vi "Get Error Details from Error Cluster.vi"(11 "error":errorcluster) -> (1 "Message":string, 2 "Call Chain":string, 3 "Source":string)   [LabVIEW 2013, in "JUnit for Azure Pipelines.lvclass"]
uses:
  JUnit for Azure Pipelines.lvclass
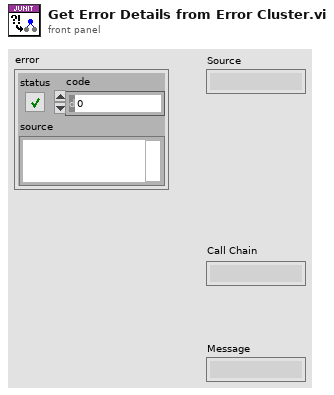
[diagram p1: front panel]
types:
  T1 = typedef "TagReturnType.ctl" = enum16{"No Tag", "<err>", "<append>"}
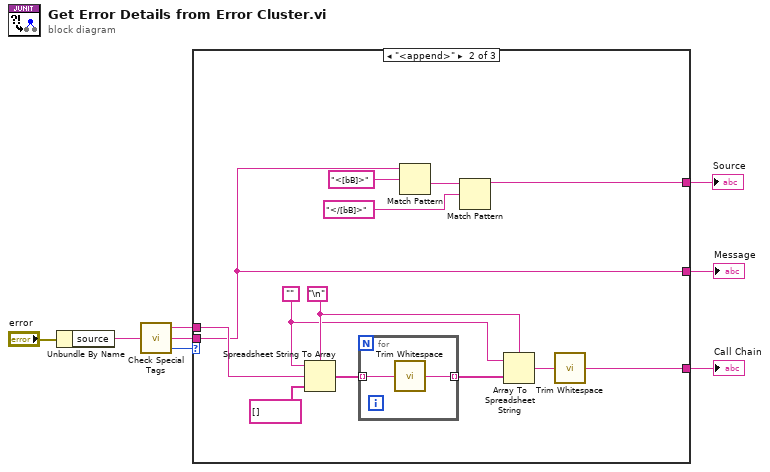
[diagram p0: block diagram]
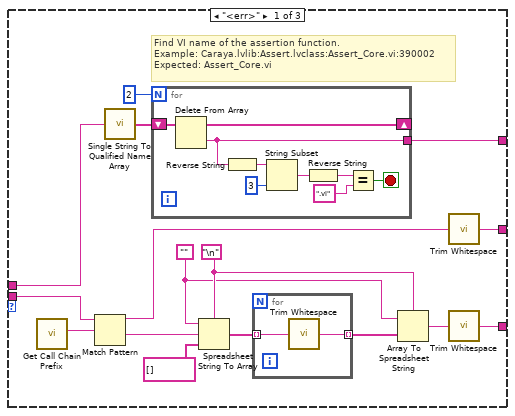
[diagram p2: hidden frame]
diagram:
  n1 = Unbundle By Name("error") -> ("source"=w1:string)
  n2 = call <vilib>:"Check Special Tags.vi"("source"=w1) -> ("Before Tag (source)"=w4:string, "After Tag (special data)"=w6:string, "Tag Found?"=w2:T1)
  n3 = case shown="\"<append>\"" w2 {
    tunnel: [w18 w41 _] -> w8
    tunnel: w6 -> [w17 w36 _]
    tunnel: [w13 w36 _] -> w5
    tunnel: w4 -> [w12 w42 _]
    tunnel: [w9 w37 _] -> w3
    frame "<err>" {
      w19 = ""
      w20 = "\n"
      # "Find VI name of the assertion function.\nExample: Caraya.lvlib:Assert.lvclass:Assert_Core.vi:390002\nExpected: Assert_Core.vi"
      n4 = call "Get Call Chain Prefix.vi"() -> ("Call Chain Prefix"=w16:string)  [unwired: 11 in]
      n5 = Match Pattern(string=w17, regular expression=w16) -> (before substring=w14:string, after substring=w15:string)  [unwired: 1 in, 2 out]
      n6 = call <vilib>:"Single String To Qualified Name Array.vi"("Fully Qualified String"=w12) -> ("Fully Qualified Array"=w11:string[])
      n7 = for {
        N: 2 -> [_]
        shift-right: [w32] -> _
        shift-left: w11 -> [w33]
        tunnel: [w25] -> w9
        stop <- w26 stop-if-true
        n8 = Delete From Array(array=w33) -> (deleted portion=w25:string, array with subset deleted=w32:string[])  [unwired: 2 in]
        n9 = Reverse String(1:w25) -> (0:w31:string)
        n10 = String Subset(string=w31, length (rest)=3 ("length (rest)")) -> (substring=w29:string)  [unwired: 1 in]
        n11 = Reverse String(1:w29) -> (0:w28:string)
        n12 = Equal?(x=w28, y=".vi") -> (x = y?=w26:bool)
      }
      n13 = Spreadsheet String To Array(delimiter (Tab)=w20, format string=w19, spreadsheet string=w15, array type (2D Dbl)=string[] []) -> (array=w23:string[])
      n14 = for {
        tunnel: [w35] -> w22 mode=indexing
        tunnel: w23 -> [w34] mode=indexing
        n15 = call <vilib>:"Trim Whitespace.vi"("string"=w34) -> ("trimmed string"=w35:string)  [unwired: 1 in]
      }
      n16 = Array To Spreadsheet String(delimiter (Tab)=w20, array=w22, 3:w19) -> (spreadsheet string=w21:string)
      n17 = call <vilib>:"Trim Whitespace.vi"("string"=w14) -> ("trimmed string"=w13:string)  [unwired: 1 in]
      n18 = call <vilib>:"Trim Whitespace.vi"("string"=w21) -> ("trimmed string"=w18:string)  [unwired: 1 in]
    }
    frame "<append>" {
      w43 = ""
      w44 = "\n"
      n19 = Spreadsheet String To Array(delimiter (Tab)=w44, format string=w43, spreadsheet string=w42, array type (2D Dbl)=string[] []) -> (array=w47:string[])
      n20 = for {
        tunnel: [w50] -> w46 mode=indexing
        tunnel: w47 -> [w49] mode=indexing
        n21 = call <vilib>:"Trim Whitespace.vi"("string"=w49) -> ("trimmed string"=w50:string)  [unwired: 1 in]
      }
      n22 = Match Pattern(string=w36, regular expression="<[bB]>") -> (after substring=w38:string)  [unwired: 1 in, 3 out]
      n23 = Match Pattern(string=w38, regular expression="</[bB]>") -> (before substring=w37:string)  [unwired: 1 in, 3 out]
      n24 = Array To Spreadsheet String(delimiter (Tab)=w44, array=w46, 3:w43) -> (spreadsheet string=w45:string)
      n25 = call <vilib>:"Trim Whitespace.vi"("string"=w45) -> ("trimmed string"=w41:string)  [unwired: 1 in]
    }
    frame "No Tag" {
    }
  }
  "Call Chain" <- w8
  "Message" <- w5
  "Source" <- w3
